vi "MiladiToShamsi.vi"(1 "Gregorian(Miladi) Date":string) -> (0 "Jalali(Shamsi) Date":string)   [LabVIEW 2015]
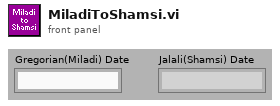
[diagram p1: front panel]
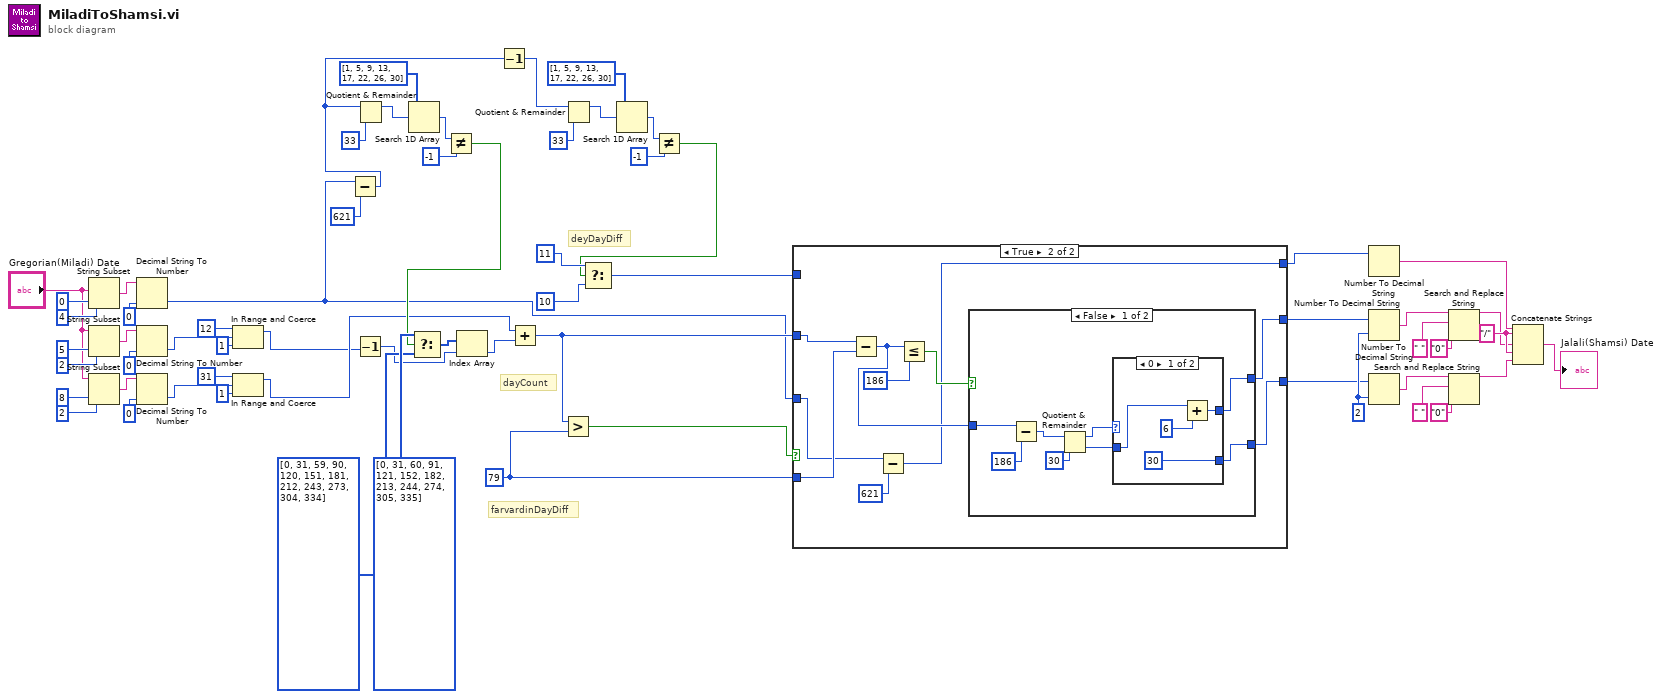
[diagram p0: block diagram]
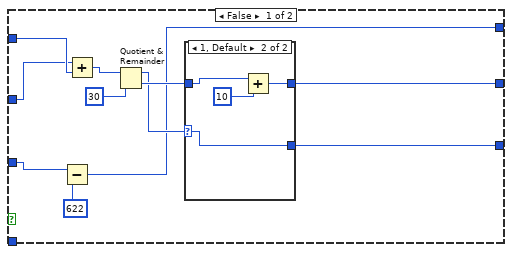
[diagram p2: hidden frame]
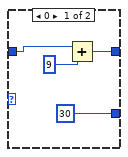
[diagram p3: hidden frame]
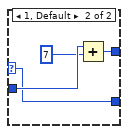
[diagram p4: hidden frame]
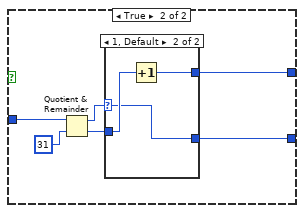
[diagram p5: hidden frame]
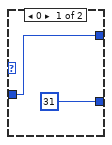
[diagram p6: hidden frame]
diagram:
  w42 = u16 79
  w56 = "/" ("string")
  w63 = u8 2 ("width (-)")
  # "farvardinDayDiff"
  # "dayCount"
  # "deyDayDiff"
  n1 = String Subset(string="Gregorian(Miladi) Date", offset (0)=0, length (rest)=4 ("length (rest)")) -> (substring=w16:string)
  n2 = String Subset(string="Gregorian(Miladi) Date", offset (0)=5, length (rest)=2 ("length (rest)")) -> (substring=w15:string)
  n3 = String Subset(string="Gregorian(Miladi) Date", offset (0)=8, length (rest)=2 ("length (rest)")) -> (substring=w14:string)
  n4 = Decimal String To Number(string=w16, default (0L)=u16 0) -> (number=w3:u16)  [unwired: 1 in, 1 out]
  n5 = Decimal String To Number(string=w15, default (0L)=u16 0) -> (number=w10:u16)  [unwired: 1 in, 1 out]
  n6 = Decimal String To Number(string=w14, default (0L)=u16 0) -> (number=w5:u16)  [unwired: 1 in, 1 out]
  n7 = In Range and Coerce(upper limit=u16 12, x=w10, lower limit=u16 1) -> (coerced(x)=w1:u16)  [unwired: 1 out]
  n8 = In Range and Coerce(upper limit=u16 31, x=w5, lower limit=u16 1) -> (coerced(x)=w2:u16)  [unwired: 1 out]
  n9 = Subtract(x=w3, y=u16 621) -> (x-y=w31:u16)
  n10 = Decrement(x=w1) -> (x-1=w49:u16)
  n11 = Quotient & Remainder(x=w31, y=u16 33) -> (x-y*floor(x/y)=w37:u16)  [unwired: 1 out]
  n12 = Search 1D Array(1D array=u16[] [1, 5, 9, 13, 17, 22, 26, 30], element=w37) -> (index of element=w35:i32)  [unwired: 1 out]
  n13 = Not Equal?(x=w35, y=-1) -> (x != y?=w32:bool)
  n14 = Select(t=u16[] [0, 31, 60, 91, 121, 152, 182, 213, 244, 274, 305, 335], s=w32, f=u16[] [0, 31, 59, 90, 120, 151, 181, 212, 243, 273, 304, 334]) -> (s? t:f=w50:u16[])
  n15 = Index Array(array=w50, index=w49) -> (element=w46:u16)
  n16 = Decrement(x=w31) -> (x-1=w25:u16)
  n17 = Add(x=w2, y=w46) -> (x+y=w44:u16)
  n18 = Greater?(x=w44, y=w42) -> (0:w45:bool)
  n19 = Quotient & Remainder(x=w25, y=u16 33) -> (x-y*floor(x/y)=w29:u16)  [unwired: 1 out]
  n20 = Search 1D Array(1D array=u16[] [1, 5, 9, 13, 17, 22, 26, 30], element=w29) -> (index of element=w27:i32)  [unwired: 1 out]
  n21 = Not Equal?(x=w27, y=-1) -> (x != y?=w24:bool)
  n22 = Select(t=u16 11, s=w24, f=u16 10) -> (s? t:f=w43:u16)
  n23 = case shown="True" w45 {
    tunnel: w44 -> [w71 w92]
    tunnel: w43 -> [w74 _]
    tunnel: w3 -> [w68 w86]
    tunnel: w42 -> [_ w91]
    tunnel: [w66 w85] -> w41
    tunnel: [w65 w84] -> w40
    tunnel: [w64 w83] -> w39
    frame False {
      n24 = Subtract(x=w68, y=u16 622) -> (x-y=w66:u16)
      n25 = Add(x=w71, y=w74) -> (x+y=w73:u16)
      n26 = Quotient & Remainder(x=w73, y=u16 30) -> (x-y*floor(x/y)=w69:u16, floor(x/y)=w70:u16)
      n27 = case shown="1, Default" w69 {
        selector: w69 -> [_ w79]
        tunnel: w70 -> [w78 w81]
        tunnel: [w76 w80] -> w65
        tunnel: [u16 30 ("y") w79] -> w64
        frame 0 {
          n28 = Add(x=w78, y=u16 9) -> (x+y=w76:u16)
        }
        frame 1, Default {
          n29 = Add(x=w81, y=u16 10) -> (x+y=w80:u16)
        }
      }
    }
    frame True {
      n30 = Subtract(x=w92, y=w91) -> (x-y=w88:u16)
      n31 = Subtract(x=w86, y=u16 621) -> (x-y=w85:u16)
      n32 = Less Or Equal?(x=w88, y=u16 186) -> (x <= y?=w89:bool)
      n33 = case shown="False" w89 {
        tunnel: w88 -> [w100 w114]
        tunnel: [w94 w110] -> w84
        tunnel: [w93 w109] -> w83
        frame False {
          n34 = Subtract(x=w100, y=u16 186) -> (x-y=w98:u16)
          n35 = Quotient & Remainder(x=w98, y=u16 30) -> (x-y*floor(x/y)=w96:u16, floor(x/y)=w95:u16)
          n36 = case shown="0" w96 {
            selector: w96 -> [_ w105]
            tunnel: w95 -> [w103 w107]
            tunnel: [u16 30 ("y") w105] -> w93
            tunnel: [w101 w108] -> w94
            frame 0 {
              n37 = Add(x=w103, y=u16 6) -> (x+y=w101:u16)
            }
            frame 1, Default {
              n38 = Add(x=w107, y=u16 7) -> (x+y=w108:u16)
            }
          }
        }
        frame True {
          n39 = Quotient & Remainder(x=w114, y=u16 31) -> (x-y*floor(x/y)=w113:u16, floor(x/y)=w112:u16)
          n40 = case shown="1, Default" w113 {
            selector: w113 -> [_ w117]
            tunnel: w112 -> [w116 w119]
            tunnel: [w116 w118] -> w110
            tunnel: [u16 31 ("y") w117] -> w109
            frame 0 {
            }
            frame 1, Default {
              n41 = Increment(x=w119) -> (x+1=w118:u16)
            }
          }
        }
      }
    }
  }
  n42 = Number To Decimal String(number=w41) -> (decimal integer string=w23:string)  [unwired: 1 out]
  n43 = Number To Decimal String(number=w40, width (-)=w63) -> (decimal integer string=w58:string)
  n44 = Number To Decimal String(number=w39, width (-)=w63) -> (decimal integer string=w57:string)
  n45 = Search and Replace String(input string=w58, search string=" ", replace string="0" ("replace string (\"\")")) -> (result string=w55:string)  [unwired: 5 in, 3 out]
  n46 = Search and Replace String(input string=w57, search string=" ", replace string="0" ("replace string (\"\")")) -> (result string=w54:string)  [unwired: 5 in, 3 out]
  n47 = Concatenate Strings(w23, w56, w55, w56, w54) -> (→"Jalali(Shamsi) Date":string)
